vi "Set Progress Property.vi"(8 "error in (no error)":errorcluster, 9 "Minimum":dbl, 10 "Maximum":dbl=100.0, 11 "UI_ProgressBar in":refnum<class "UI_ProgressDlg.lvclass">) -> (0 "error out":errorcluster, 3 "UI_ProgressBar out":refnum<class "UI_ProgressDlg.lvclass">)   [LabVIEW 2014, in "UI_ProgressDlg.lvlib" / "UI_ProgressDlg.lvclass"]
uses:
  UI_ProgressDlg.lvclass
  <vilib>/Utility/miscctls.llb/LVRangeTypeDef.ctl
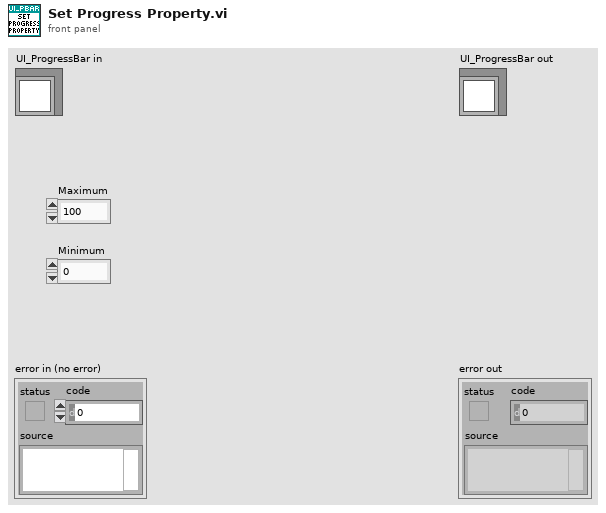
[diagram p1: front panel]
types:
  T1 = typedef "LVRangeTypeDef.ctl" = cluster{"Minimum":dbl, "Maximum":dbl, "Increment":dbl, "Minor Increment":dbl, "Start":dbl}
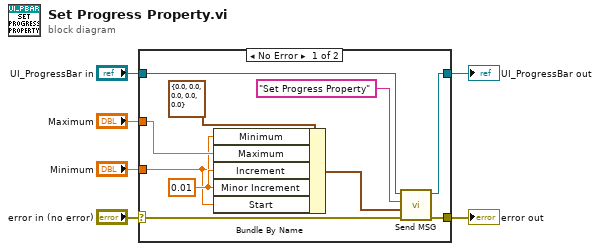
[diagram p0: block diagram]
diagram:
  n1 = case shown="No Error" "error in (no error)" {
    selector: "error in (no error)" -> [w12 w18]
    tunnel: [w11 w18] -> w5
    tunnel: [w13 w17] -> w3
    tunnel: "UI_ProgressBar in" -> [w14 w17]
    tunnel: "Maximum" -> [w15 _]
    tunnel: "Minimum" -> [w8 _]
    frame No Error {
      w9 = 0.01 ("Increment")
      n2 = Bundle By Name(cluster=T1 {"Minimum"=0.0, "Maximum"=0.0, "Increment"=0.0, "Minor Increment"=0.0, "Start"=0.0} ("Scale.Range"), "Minimum"=w8, "Maximum"=w15, "Increment"=w9, "Minor Increment"=w9, "Start"=w8) -> (w7:T1)
      n3 = call "Send MSG.vi"("error in (no error)"=w12, "msg value"=w7, "msg"="Set Progress Property", "UI_ProgressBar in"=w14) -> ("error out"=w11:errorcluster, "UI_ProgressBar out"=w13:refnum<class "UI_ProgressDlg.lvclass">)  [unwired: 6 in]
    }
    frame Error {
    }
  }
  "error out" <- w5
  "UI_ProgressBar out" <- w3
